vi "Calculate Shooter Speed.vi"(11 "Shoot":bool) -> (3 "Shooter Speed out":dbl)   [LabVIEW 2020]
uses:
  Robot Global Data.vi
  <vilib>/Rock Robotics/Network Tables/NT Read Numeric Array.vi
  2017 Swerve Code/Swerve Global Variables.vi
panel:
  in  "speed lookup table":dbl[](array[numeric])
  out "Raspberry pi info":dbl[](array[numeric])
  in  "Default Shooter Speed in":dbl=3100.0
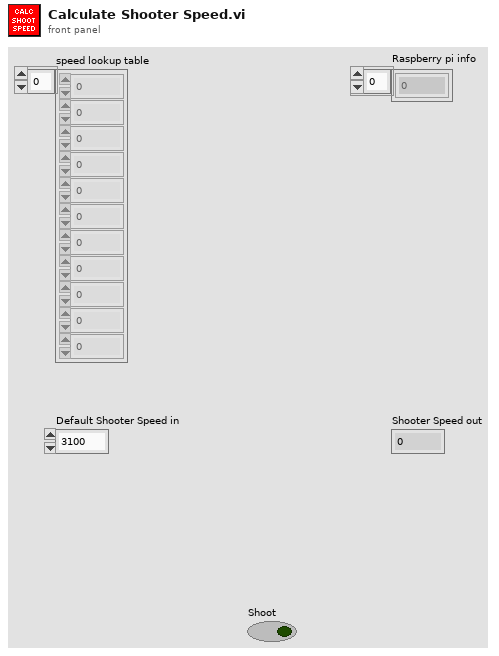
[diagram p1: front panel]
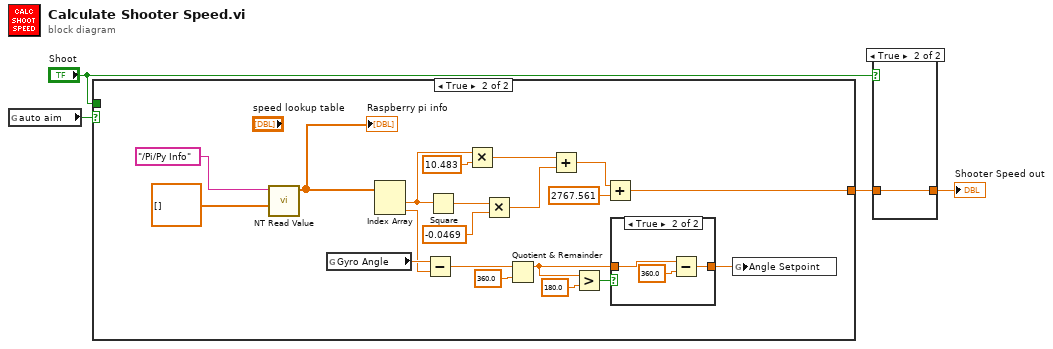
[diagram p0: block diagram]
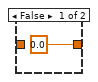
[diagram p2: hidden frame]
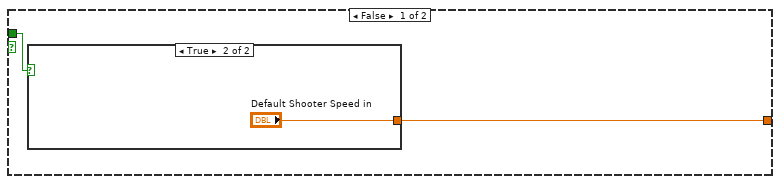
[diagram p3: hidden frame]
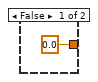
[diagram p4: hidden frame]
diagram:
  n1 = global read "Robot Global Data.vi" "auto aim"() -> (w1:bool)
  n2 = case shown="True" w1 {
    tunnel: [w5 w9] -> w2
    tunnel: "Shoot" -> [w6 _]
    frame False {
      n3 = case shown="True" w6 {
        tunnel: [0.0 "Default Shooter Speed in"] -> w5
        frame False {
        }
        frame True {
        }
      }
    }
    frame True {
      n4 = call-poly <vilib>:"NT Read Value.vi"("Default Value"=dbl[] [], "Name"="/Pi/Py Info") -> ("Numeric Array"=w26:dbl[])  [unwired: 8 in, 1 out]
      "Raspberry pi info" <- w26
      n5 = global read "Swerve Global Variables.vi" "Gyro Angle"() -> (w25:dbl)
      n6 = Index Array(array=w26) -> (element #1=w14:dbl, element #2=w18:dbl)  [unwired: 2 in]
      n7 = Subtract(x=w25, y=w18) -> (x-y=w24:dbl)
      n8 = Square(x=w14) -> (x^2=w17:dbl)
      n9 = Multiply(x=w14, y=10.483) -> (x*y=w13:dbl)
      n10 = Multiply(x=w17, y=-0.0469) -> (x*y=w12:dbl)
      n11 = Quotient & Remainder(x=w24, y=360.0) -> (x-y*floor(x/y)=w20:dbl)  [unwired: 1 out]
      n12 = Add(x=w13, y=w12) -> (x+y=w10:dbl)
      n13 = Greater?(x=w20, y=180.0) -> (0:w21:bool)
      n14 = Add(x=w10, y=2767.561) -> (x+y=w9:dbl)
      n15 = case shown="True" w21 {
        tunnel: [w29 w30] -> w19
        tunnel: w20 -> [w29 w32]
        frame False {
        }
        frame True {
          n16 = Subtract(x=w32, y=360.0) -> (x-y=w30:dbl)
        }
      }
      n17 = global write "Robot Global Data.vi" "Angle Setpoint"(w19) -> ()
    }
  }
  n18 = case shown="True" "Shoot" {
    tunnel: [0.0 w34] -> w3
    tunnel: w2 -> [_ w34]
    frame False {
    }
    frame True {
    }
  }
  "Shooter Speed out" <- w3
